vi "addTest.vi"(8 "error in (no error)":errorcluster, 10 "test":refnum<class>, 11 "TestSuite in":refnum<class "TestSuite.lvclass">) -> (0 "error out":errorcluster, 3 "TestSuite out":refnum<class "TestSuite.lvclass">)   [LabVIEW 2019, in "TestSuite.lvclass"]
doc: "Adds a 'test' to a TestSuite object. 'test' can be a TestCase or TestSuite object."
uses:
  TestSuite.lvclass
  TestCase/TestCase.lvclass
  TestSuite.lvclass/TestSuite.ctl
  Libraries/VITesterUtilities.lvlib
panel:
  # "JKI VI Tester for LabVIEW\nhttp://jkisoft.com/vi-tester\nCopyright (C) 2007-2009, JKI <info@jkisoft.com>\nALL RIGHTS RESERVED"
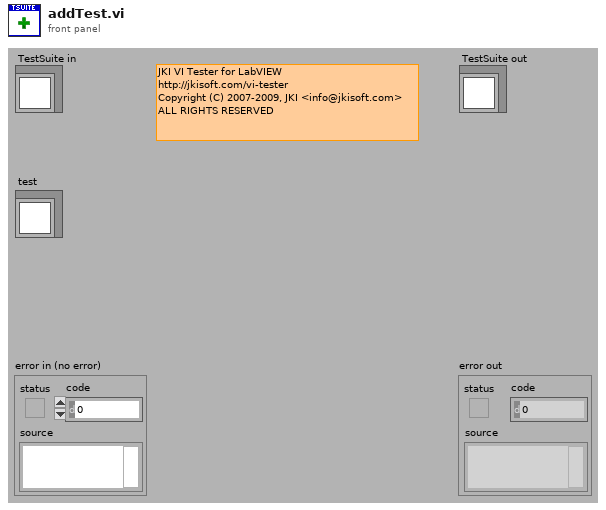
[diagram p1: front panel]
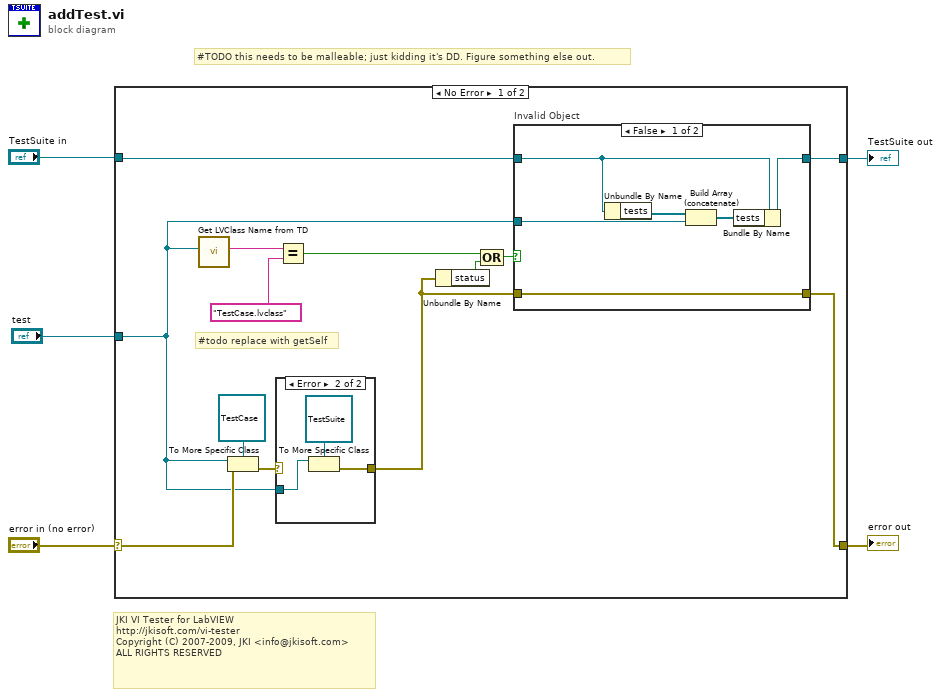
[diagram p0: block diagram]
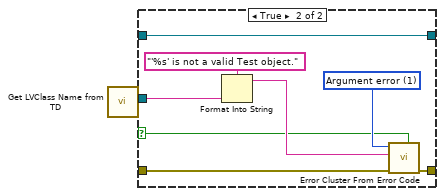
[diagram p2: hidden frame]
diagram:
  # "#TODO this needs to be malleable; just kidding it's DD. Figure something else out."
  # "JKI VI Tester for LabVIEW\nhttp://jkisoft.com/vi-tester\nCopyright (C) 2007-2009, JKI <info@jkisoft.com>\nALL RIGHTS RESERVED"
  n1 = case shown="No Error" "error in (no error)" {
    selector: "error in (no error)" -> [w14 w39]
    tunnel: [w13 w39] -> w4
    tunnel: [w17 w38] -> w2
    tunnel: "TestSuite in" -> [w18 w38]
    tunnel: "test" -> [w12 _]
    frame No Error {
      # "#todo replace with getSelf"
      n2 = call "Get LVClass Name from TD.vi"("Variant"=w12) -> ("LVClass Name"=w10:string)  [unwired: 9 in, 1 out]
      n3 = To More Specific Class(target class=refnum<class "TestCase.lvclass"> refnum ("TestCase.lvclass"), reference=w12, error in=w14) -> (error out=w15:errorcluster)  [unwired: 1 out]
      n4 = case shown="Error" w15 {
        selector: w15 -> [w34 _]
        tunnel: w12 -> [_ w37]
        tunnel: [w34 w35] -> w9
        frame No Error {
        }
        frame Error {
          n5 = To More Specific Class(target class=refnum<class "TestSuite.lvclass"> refnum ("TestSuite.lvclass"), reference=w37) -> (error out=w35:errorcluster)  [unwired: 1 in, 1 out]
        }
      }
      n6 = Equal?(x=w10, y="TestCase.lvclass") -> (x = y?=w6:bool)
      n7 = Unbundle By Name(w9) -> ("status"=w11:bool)
      n8 = Compound Arithmetic op=OR(w6, w11) -> (w8:bool)
      n9 = case "Invalid Object" shown="False" w8 {
        selector: w8 -> [_ w25]
        tunnel: w18 -> [w23 w28]
        tunnel: [w22 w28] -> w17
        tunnel: w12 -> [w20 w31]
        tunnel: [w19 w33] -> w13
        tunnel: w9 -> [w19 w26]
        frame False {
          n10 = Unbundle By Name(w23) -> ("tests"=w24:refnum<class>[])
          n11 = Build Array (concatenate)(w24, w20) -> (w21:refnum<class>[])
          n12 = Bundle By Name(cluster=w23, "tests"=w21) -> (w22:refnum<class "TestSuite.lvclass">)
        }
        frame True {
          w32 = 1 items=["No error", "Argument error", "Memory is full", "Out of zone", "End of file", "File already open", "Generic file I/O error", "File not found", "File permission error", "Disk is full", "Duplicate path", "Too many files open", "System feature not enabled", "Resource file not found", "Cannot add resource", "Resource not found", "Image not found", "Image memory error", "Pen does not exist", "Config type invalid", "Config token not found", "Config parse error", "Config memory error", "Bad external code format", "Bad external code offset", "External code not present", "Null window", "Destroy window error", "Null menu", "Print aborted", "Bad print record", "Print driver error", "Windows error during printing", "Memory error during printing", "Print dialog error", "Generic print error", "Invalid device refnum", "Device not found", "Device parameter error", "Device unit error", "Cannot open device", "Device call aborted", "Generic error", "Cancelled by user", "Object ID too low", "Object ID too high", "Object not in heap", "Unknown heap", "Unknown object (invalid DefProc)", "Unknown object (DefProc not in table)", "Message out of range", "Invalid (null) method", "Unknown message", "Manager call not supported", "Bad address", "Network operation in progress", "Network operation timed out", "Connection is busy", "Network attribute not supported", "Network error", "Address in use", "System out of memory", "Connection aborted", "Connection refused", "Not connected", "Already connected", "Connection closed", "Initialization error (interapplication manager)", "Bad occurrence", "Wait on unbound occurrence handler", "Occurrence queue overflow", "Datalog type conflict", "Unused", "Unrecognized type (interapplication manager)", "Memory corrupt", "Failed to make temporary DLL", "Old CIN version", "Drag socket not found", "Failed to load drop-object", "Failed to register OLE object", "Failed to release OLE object", "Format specifier type mismatch", "Unknown format specifier", "Too few format specifiers", "Too many format specifiers", "Scan failed", "Newer CIN version", "Error converting to variant", "Runtime menu error", "Password tampered", "Variant attribute not found", "Incompatible variant data type", "Event data is not available", "Event Store is not present", "Occurrence is not found", "Event Queue is not created", "Event info is not available", "Refnum passed is NULL", "Error retrieving Class GUID", "Error retrieving CoClass GUID", "Error retrieving TypeLib GUID.", "Bad built application magic bytes.", "Specific driver is different from the specific driver associated with the Logical Name.", "There is no session opened to the class driver.", "Max Error", "MAX - Error with config objects", "MAX - Error loading configuration", "MAX - Group not supported"]
          n13 = call "Get LVClass Name from TD.vi"("Variant"=w31) -> ("LVClass Name"=w29:string)  [unwired: 9 in, 1 out]
          n14 = Format Into String(format string="'%s' is not a valid Test object.", w29) -> (resulting string=w30:string)  [unwired: 2 in, 1 out]
          n15 = call <vilib>:"Error Cluster From Error Code.vi"("is warning? (False)"=w25, "error in (no error)"=w26, "error message (\"\")"=w30, "error code (0)"=w32) -> ("error out"=w33:errorcluster)  [unwired: 5 in]
        }
      }
    }
    frame Error {
    }
  }
  "error out" <- w4
  "TestSuite out" <- w2
